vi "AUTON_Straight_&_Turn.vi"(9 "Power":dbl, 10 "Current Heading":dbl, 11 "Desired Heading":dbl) -> (2 "Right Drive":dbl, 3 "Left Drive":dbl)   [LabVIEW 2012]
panel:
  out "Delta heading":dbl
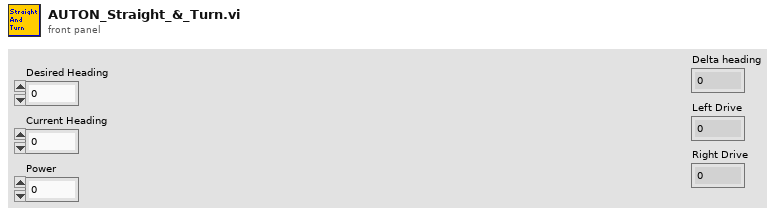
[diagram p1: front panel]
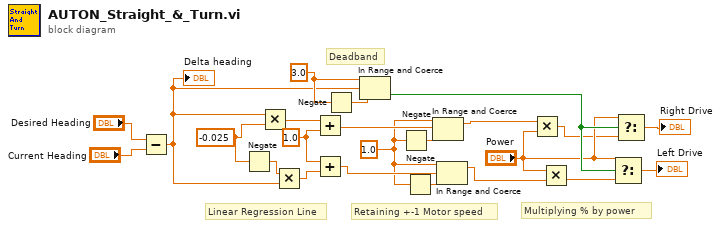
[diagram p0: block diagram]
diagram:
  w1 = 1.0 ("upper limit")
  w21 = 3.0 ("upper limit")
  w14 = 1.0 ("y")
  w17 = -0.025 ("y")
  # "Deadband"
  # "Multiplying % by power"
  # "Retaining +-1 Motor speed"
  # "Linear Regression Line"
  n1 = Subtract(x="Desired Heading", y="Current Heading") -> (x-y=w16:dbl)
  "Delta heading" <- w16
  n2 = Negate(x=w17) -> (-x=w18:dbl)
  n3 = Multiply(x=w16, y=w17) -> (x*y=w23:dbl)
  n4 = Multiply(x=w18, y=w16) -> (x*y=w15:dbl)
  n5 = Add(x=w23, y=w14) -> (x+y=w12:dbl)
  n6 = Add(x=w14, y=w15) -> (x+y=w10:dbl)
  n7 = Negate(x=w21) -> (-x=w22:dbl)
  n8 = In Range and Coerce(upper limit=w21, x=w16, lower limit=w22) -> (In Range?=w9:bool)  [unwired: 1 out]
  n9 = Negate(x=w1) -> (-x=w13:dbl)
  n10 = Negate(x=w1) -> (-x=w11:dbl)
  n11 = In Range and Coerce(upper limit=w1, x=w12, lower limit=w13) -> (coerced(x)=w5:dbl)  [unwired: 1 out]
  n12 = In Range and Coerce(upper limit=w1, x=w10, lower limit=w11) -> (coerced(x)=w6:dbl)  [unwired: 1 out]
  n13 = Multiply(x=w5, y="Power") -> (x*y=w3:dbl)
  n14 = Multiply(x="Power", y=w6) -> (x*y=w2:dbl)
  n15 = Select(t="Power", s=w9, f=w2) -> (s? t:f=→"Left Drive":dbl)
  n16 = Select(t="Power", s=w9, f=w3) -> (s? t:f=→"Right Drive":dbl)
